vi "TestBenchVariables.vi"() -> ()   [LabVIEW 2015, in "TestBench.lvlib"]
uses:
  TestBench.lvlib
panel:
  in  "Voltage PV":dbl
  out "Reset":bool
  out "Unconfirmed Error?":bool
  in  "Error":errorcluster
  out "Quit?":bool
  out "Motor Enable?":bool
  in  "RPM PV":dbl
  in  "Current PV":dbl
  in  "Serwo Angle SP":dbl
  in  "Voltage SP":dbl
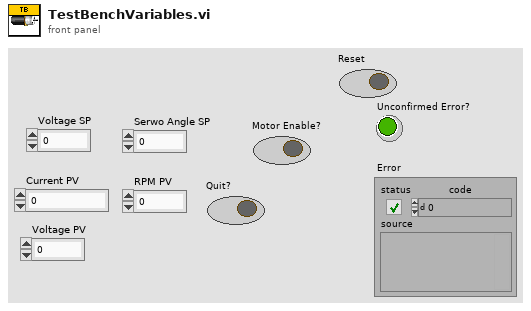
[diagram p1: front panel]
diagram:
